vi "Read Colors [2].vi"(8 "error in (no error)":errorcluster, 11 "MultiSegmentPipe.lvclass in":refnum<class "MultiSegmentPipe.lvclass">) -> (0 "error out":errorcluster, 2 "Colors[2]":cluster{u32, u32}[](array[cluster]), 3 "MultiSegmentPipe.lvclass out":refnum<class "MultiSegmentPipe.lvclass">)   [LabVIEW 2015, in "MultiSegmentPipe.lvclass"]
uses:
  MultiSegmentPipe.lvclass
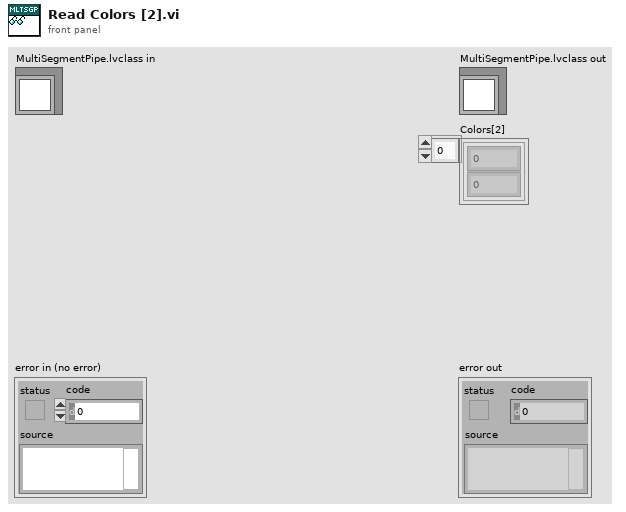
[diagram p1: front panel]
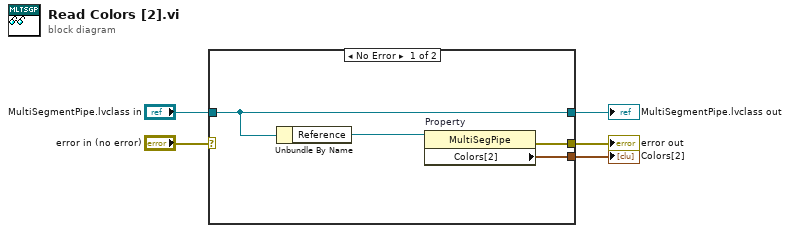
[diagram p0: block diagram]
diagram:
  n1 = case shown="No Error" "error in (no error)" {
    selector: "error in (no error)" -> [_ w11]
    tunnel: [w8 w11] -> w4
    tunnel: [w7 w10] -> w2
    tunnel: "MultiSegmentPipe.lvclass in" -> [w7 w10]
    tunnel: [w9 _] -> w1
    frame No Error {
      n2 = Unbundle By Name(w7) -> ("Reference"=w6:refnum<vi>)
      n3 = property on="Property" class="MultiSegPipe"(reference=w6) -> (error out=w8:errorcluster, "Colors[2]"=w9:cluster{u32, u32}[])  [unwired: 1 in, 1 out]
    }
    frame Error {
    }
  }
  "error out" <- w4
  "MultiSegmentPipe.lvclass out" <- w2
  "Colors[2]" <- w1
